vi "Read SnP File (SnP).vi"(0 "SnP File Path":path, 5 "Swap Ports (False)":bool, 11 "Error In":errorcluster) -> (4 "S-parameters":cdb[][](array[numeric]) format="%#.6g", 6 "Frequencies (Hz)":dbl[](array[numeric]), 8 "Z0 (Ohm)":cdb, 15 "Error Out":errorcluster)   [LabVIEW 2023, in "NI_HFNetworkAnalysis.lvlib"]
doc: "Reads n-Port S-parameters from the specified file assuming Touchstone File Format specifications.\n\n<b>Known limitation :</b>\nSupport for S-parameter data only."
uses:
  NI_HFNetworkAnalysis.lvlib
  C:/srd-semi-rfcal-software/AuxTools/STSRFFixtureCharactUtility/Source/Code Modules/Fixture/Dependencies/HFNetworkAnalysis/Support Files/NACE.Utils.Data.dll
  Support Files/NACE.Utils.Data.dll
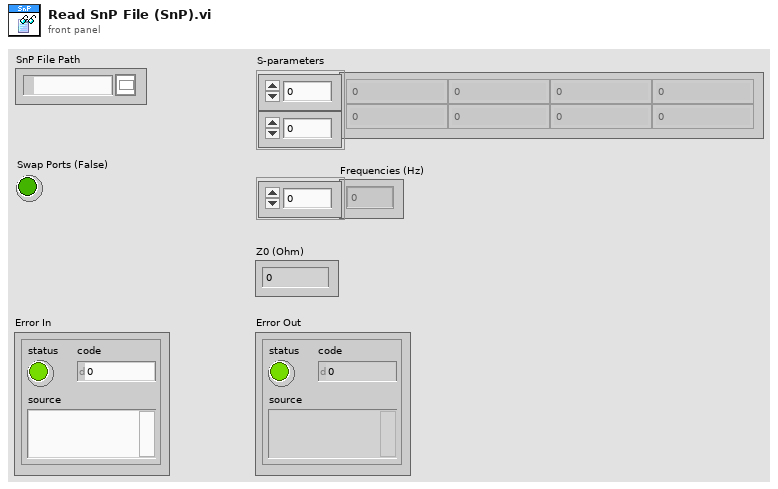
[diagram p1: front panel]
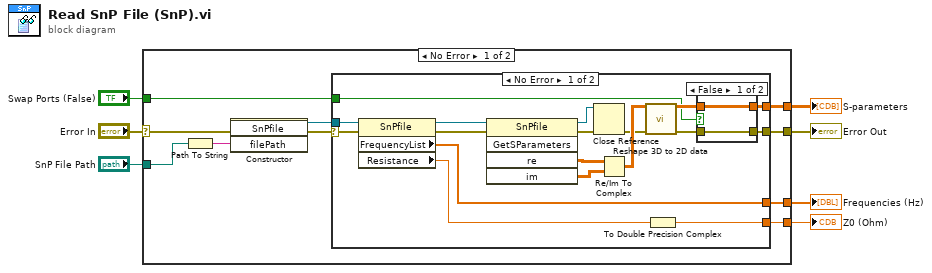
[diagram p0: block diagram]
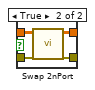
[diagram p2: hidden frame]
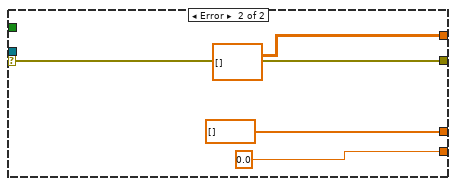
[diagram p3: hidden frame]
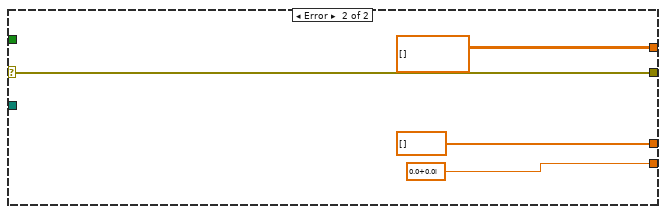
[diagram p4: hidden frame]
diagram:
  n1 = case shown="No Error" "Error In" {
    selector: "Error In" -> [w13 w49]
    tunnel: [w12 w49] -> w6
    tunnel: "SnP File Path" -> [w14 _]
    tunnel: [w11 cdb[][] [] ("Parameters Out (2D)")] -> w4
    tunnel: [w10 dbl[] [] ("FrequencyList")] -> w3
    tunnel: [w9 cdb 0.0+0.0i ("Resistance")] -> w2
    tunnel: "Swap Ports (False)" -> [w8 _]
    frame No Error {
      n2 = Path To String(path=w14) -> (string=w15:string)
      n3 = constructor class="SnPfile"(error in=w13, "filePath"=w15) -> (reference out=w16:refnum<k24>, error out=w17:errorcluster)  [unwired: 2 in, 2 out]
      n4 = case shown="No Error" w17 {
        selector: w17 -> [w34 w42]
        tunnel: w16 -> [w35 _]
        tunnel: [w28 dbl[] [] ("FrequencyList")] -> w10
        tunnel: [w27 0.0 ("Resistance")] -> w9
        tunnel: [w21 dbl[][] [] ("FrequencyList")] -> w11
        tunnel: [w24 w42] -> w12
        tunnel: w8 -> [w18 _]
        frame No Error {
          n5 = property class="SnPfile"(reference=w35, error in=w34) -> (reference out=w33:refnum<k24>, error out=w32:errorcluster, "FrequencyList"=w28:dbl[], "Resistance"=w29:dbl)
          n6 = invoke class="SnPfile" method="GetSParameters"(reference=w33, error in=w32) -> (reference out=w19:refnum<k24>, error out=w25:errorcluster, "re"=w31:dbl[][][], "im"=w30:dbl[][][])  [unwired: 3 in, 1 out]
          n7 = Close Reference(reference=w19, error in (no error)=w25) -> (error out=w20:errorcluster)
          n8 = Re/Im To Complex(1:w30, 2:w31) -> (0:w26:cdb[][][])
          n9 = call "Reshape 3D to 2D data.vi"("Parameters In (3D)"=w26, "Error In"=w20) -> ("Parameters Out (2D)"=w22:cdb[][], "Error Out"=w23:errorcluster)  [unwired: 12 in]
          n10 = To Double Precision Complex(1:w29) -> (0:w27:cdb)
          n11 = case shown="False" w18 {
            tunnel: [w36 w41] -> w24
            tunnel: w23 -> [w36 w40]
            tunnel: w22 -> [w37 w39]
            tunnel: [w37 w38] -> w21
            frame False {
            }
            frame True {
              n12 = call "Swap 2nPort.vi"("error in (no error)"=w40, "Parameters In (2D)"=w39) -> ("error out"=w41:errorcluster, "Parameters Out (2D)"=w38:cdb[][])  [unwired: 8 in]
            }
          }
        }
        frame Error {
        }
      }
    }
    frame Error {
    }
  }
  "Error Out" <- w6
  "S-parameters" <- w4
  "Frequencies (Hz)" <- w3
  "Z0 (Ohm)" <- w2
